vi "mult_process.vi"() -> ()   [LabVIEW 2013]
uses:
  G:/Romanova/results_cluster.ctl
  <vilib>/Utility/file.llb/Read From Spreadsheet File (DBL).vi
  <vilib>/gmath/statdist.llb/Student t Inverse CDF.vi
  <vilib>/Analysis/NI_AALBase.lvlib
  <vilib>/gmath/NI_Gmath.lvlib
panel:
  out "Промахи":dbl[](array[numeric])
  in  "Значимость":dbl
  in  "Строка форматирования":string="%_5f ± %_3f; %_2f"
  out "Результат измерений":string
  in  "Pдов":dbl=0.95
  in  "Границы НСП":dbl
  out "Результаты обработки":T1 {"Dдов рез" format="%#.4g"; "S сумм" format="%#.4g"; "К" format="%#.4g"; "Dдов случ." format="%#.4g"; "Sхср" format="%#.4g"; "S" format="%#.4g"}
  in  "Записать результат":bool
  in  "Получить данные":bool
  in  "Вычислить Dдов":bool
  out "Ряд измерений":dbl[](graph)
  in  "Стоп":bool
  in  "Вычислить оценки":bool
  in  "Путь":path caption="Путь к файлу"
  # "Обработка результатов многократных измерений"
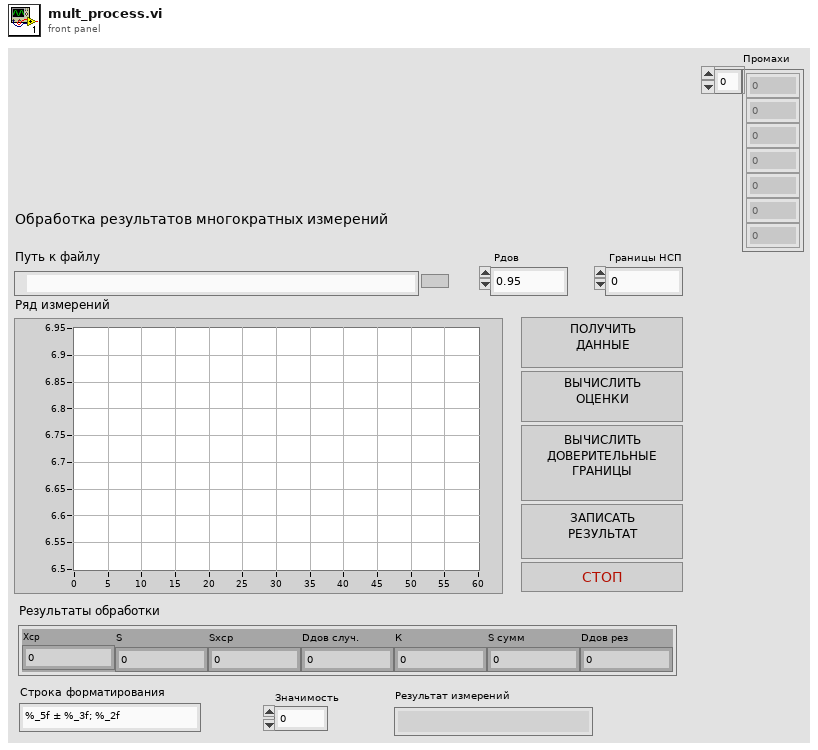
[diagram p1: front panel]
types:
  T1 = typedef "results_cluster.ctl" = cluster{"Xср":dbl, "S":dbl, "Sхср":dbl, "Dдов случ.":dbl, "К":dbl, "S сумм":dbl, "Dдов рез":dbl}
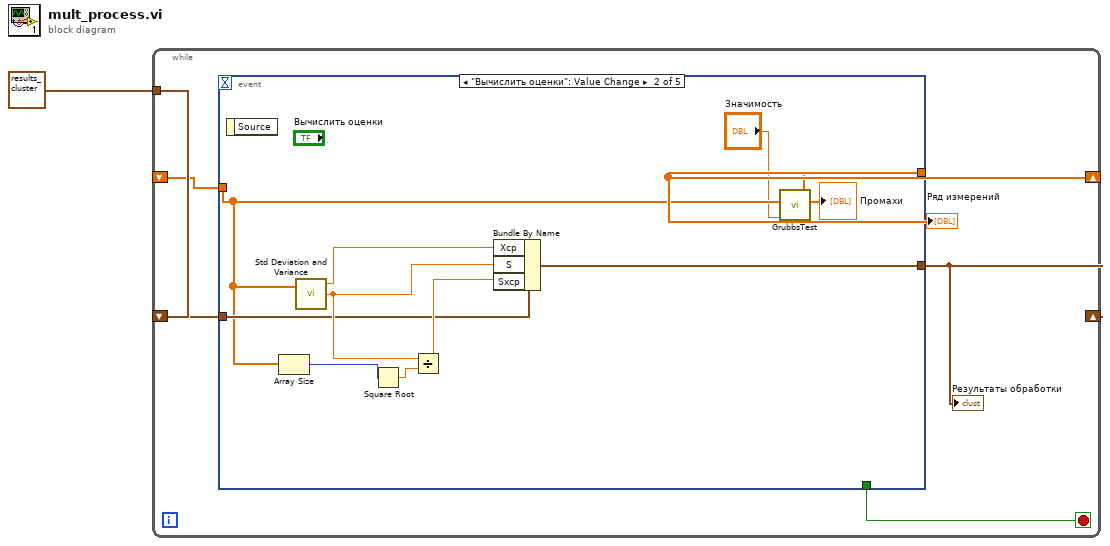
[diagram p0: block diagram]
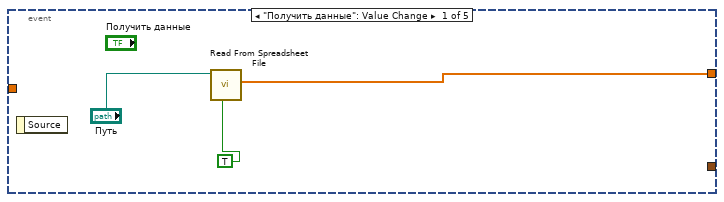
[diagram p2: hidden frame]
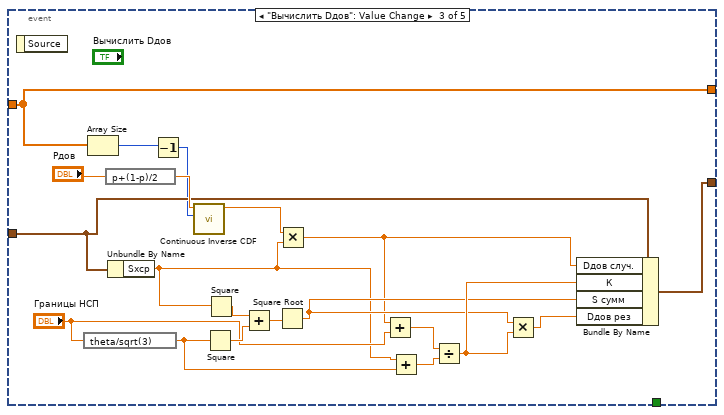
[diagram p3: hidden frame]
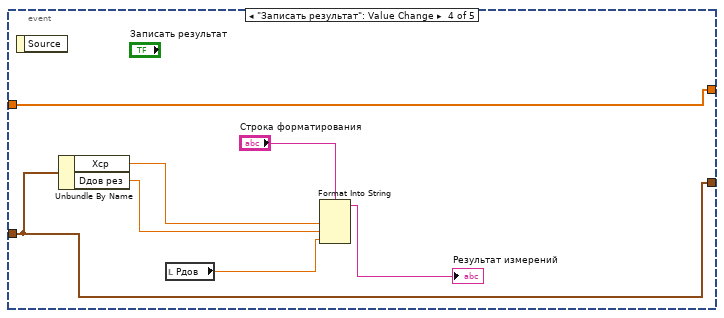
[diagram p4: hidden frame]
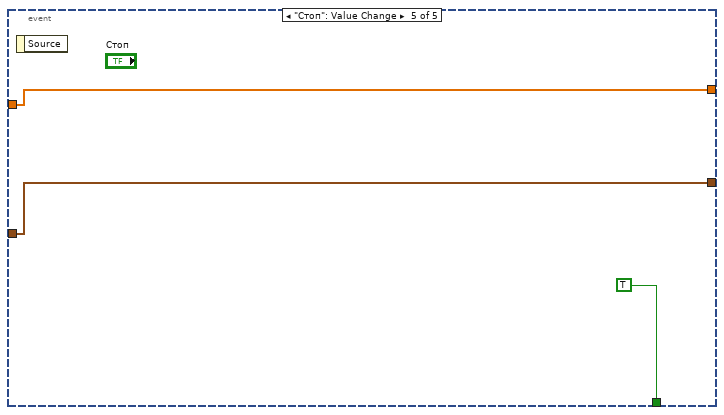
[diagram p5: hidden frame]
diagram:
  w1 = T1 {"Xср"=1.3199999999999998, "S"=0.130384048104053, "Sхср"=0.05830951894845301, "Dдов случ."=0.16189317847087023, "К"=2.43060784036949, "S сумм"=0.06506407098647712, "Dдов рез"=0.15814524106608838} ("Результаты обработки")
  n1 = while {
    shift-right: [w6] -> _
    shift-left: _ -> [w5]
    shift-right: [w3] -> _
    shift-left: w1 -> [w4]
    tunnel: w1 -> [_]
    stop <- w2 stop-if-true
    n2 = event shown="[1] \"Вычислить оценки\": Value Change" {
      selector: _ -> [_ _ _ _ _]
      dyn-events: _ -> [_ _ _ _ _]
      timeout: _ -> [_ _ _ _ _]
      tunnel: [w7 w11 w23 w41 w50] -> w6
      tunnel: w5 -> [_ w13 w23 w41 w50]
      tunnel: w4 -> [_ w14 w25 w47 w49]
      tunnel: [_ w19 w38 w47 w49] -> w3
      tunnel: [_ _ _ _ TRUE] -> w2
      event "Получить данные": Value Change {
        n3 = event-data() -> ()  [unwired: 1 in, 1 out]
        n4 = call-poly <vilib>:"Read From Spreadsheet File.vi"("transpose (no:F)"=TRUE, "file path (dialog if empty)"="Путь") -> ("first row"=w7:dbl[])  [unwired: 5 in, 4 out]
      }
      event "Вычислить оценки": Value Change {
        n5 = event-data() -> ()  [unwired: 1 in, 1 out]
        n6 = Array Size(array=w13) -> (size(s)=w18:i32)
        n7 = call <vilib>:"Std Deviation and Variance.vi"("X"=w13) -> ("mean"=w20:dbl, "standard deviation"=w16:dbl)  [unwired: 1 in, 1 out]
        n8 = Square Root(x=w18) -> (sqrt(x)=w17:dbl)
        n9 = Divide(x=w16, y=w17) -> (x/y=w15:dbl)
        n10 = Bundle By Name(cluster=w14, "Xср"=w20, "S"=w16, "Sхср"=w15) -> (w19:T1)
        n11 = call "GrubbsTest.vi"("Значимость"="Значимость", "Исходные"=w13) -> ("Промахи"=→"Промахи":dbl[], "Обработанные"=w11:dbl[])  [unwired: 2 in, 2 out]
      }
      event "Вычислить Dдов": Value Change {
        n12 = event-data() -> ()  [unwired: 1 in, 1 out]
        n13 = expression code="theta/sqrt(3)"("Границы НСП") -> (w26:dbl)
        n14 = Array Size(array=w23) -> (size(s)=w22:i32)
        n15 = expression code="p+(1-p)/2"("Pдов") -> (w39:dbl)
        n16 = Unbundle By Name(w25) -> ("Sхср"=w24:dbl)
        n17 = Decrement(x=w22) -> (x-1=w21:i32)
        n18 = call-poly <vilib>:"Continuous Inverse CDF.vi"("k degrees of freedom"=w21, "cdf(x)"=w39) -> ("x"=w34:dbl)  [unwired: 8 in, 1 out]
        n19 = Square(x=w26) -> (x^2=w36:dbl)
        n20 = Square(x=w24) -> (x^2=w37:dbl)
        n21 = Add(x=w37, y=w36) -> (x+y=w35:dbl)
        n22 = Square Root(x=w35) -> (sqrt(x)=w30:dbl)
        n23 = Multiply(x=w34, y=w24) -> (x*y=w28:dbl)
        n24 = Add(x=w28, y="Границы НСП") -> (x+y=w33:dbl)
        n25 = Add(x=w24, y=w26) -> (x+y=w32:dbl)
        n26 = Divide(x=w33, y=w32) -> (x/y=w31:dbl)
        n27 = Multiply(x=w30, y=w31) -> (x*y=w29:dbl)
        n28 = Bundle By Name(cluster=w25, "Dдов случ."=w28, "К"=w31, "S сумм"=w30, "Dдов рез"=w29) -> (w38:T1)
      }
      event "Записать результат": Value Change {
        n29 = event-data() -> ()  [unwired: 1 in, 1 out]
        n30 = Unbundle By Name(w47) -> ("Xср"=w42:dbl, "Dдов рез"=w43:dbl)
        n31 = local read "Pдов"() -> (w44:dbl)
        n32 = Format Into String(format string="Строка форматирования", w42, w43, w44) -> (resulting string=→"Результат измерений":string)  [unwired: 2 in, 1 out]
      }
      event "Стоп": Value Change {
        n33 = event-data() -> ()  [unwired: 1 in, 1 out]
      }
    }
    "Ряд измерений" <- w6
    "Результаты обработки" <- w3
  }
